vi "Merge_and_append.vi"(1 "New Row":string[](array[string]), 2 "Comments":string[](array[string]), 3 "Channel Names":string[](array[string]), 4 "Path name":path) -> (0 "File Updated?":bool)   [LabVIEW 2010]
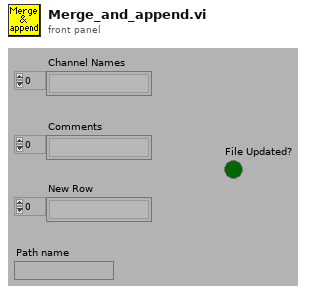
[diagram p1: front panel]
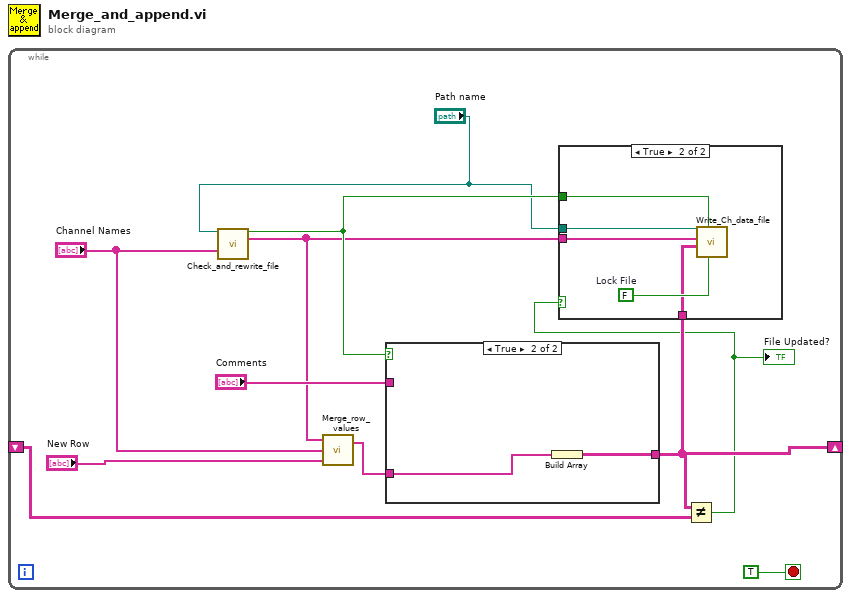
[diagram p0: block diagram]
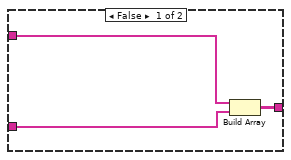
[diagram p3: hidden frame]
diagram:
  n1 = while {
    shift-right: [w3] -> _
    shift-left: _ -> [w2]
    stop <- TRUE stop-if-true
    n2 = call "Check_and_rewrite_file.vi"("Filename"="Path name", "Present Channels"="Channel Names") -> ("exists?"=w10:bool, "Merged Channels"=w9:string[])  [unwired: 2 in, 10 out]
    n3 = call "Merge_row_values.vi"("Present Row values"="New Row", "Present Channels"="Channel Names", "Desired Channels"=w9) -> ("Desired Row values"=w6:string[])  [unwired: 1 out]
    n4 = case shown="True" w10 {
      tunnel: w6 -> [w19 w21]
      tunnel: [w18 w20] -> w3
      tunnel: "Comments" -> [w17 _]
      frame False {
        n5 = Build Array(w17, w19) -> (w18:string[][])
      }
      frame True {
        n6 = Build Array(w21) -> (w20:string[][])
      }
    }
    n7 = Not Equal?(x=w3, y=w2) -> (x != y?=w1:bool)
    "File Updated?" <- w1
    n8 = case shown="True" w1 {
      tunnel: w10 -> [_ w16]
      tunnel: w9 -> [_ w15]
      tunnel: "Path name" -> [_ w14]
      tunnel: w3 -> [_ w12]
      frame False {
      }
      frame True {
        w13 = FALSE  # Lock File
        n9 = call "Write_Ch_data_file.vi"("Lock File"=w13, "exists?"=w16, "Channel Values"=w12, "Channel names"=w15, "Filename"=w14) -> ()  [unwired: 3 in, 4 out]
      }
    }
  }
